vi "Python@SetVariable(Worker)__Parameter.vi"(1 "ParamterIn":string) -> (0 "ParamterOut":string)   [LabVIEW 2020]
panel:
  in  "Session":string(combo)
  in  "PythonName":string(combo) caption="PythonName="
  in  "Section":string(combo)
  in  "ParameterName":string(combo)
  in  "Confirm":bool
  # "Python@SetVariable(Worker) $Worker$Variable(,$section,PythonName=)"
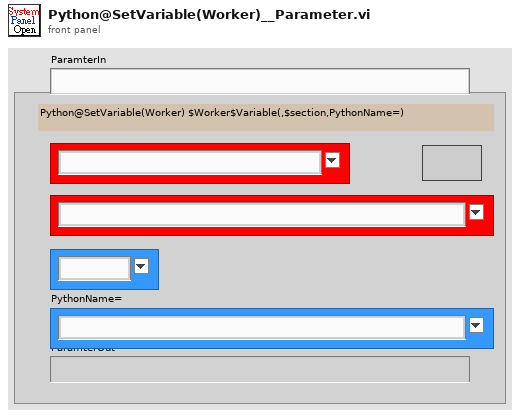
[diagram p1: front panel]
types:
  T1 = enum16{"Get", "Init", "Set", "Delete", "GetElement", "Inc", "Dec", "ReName"}
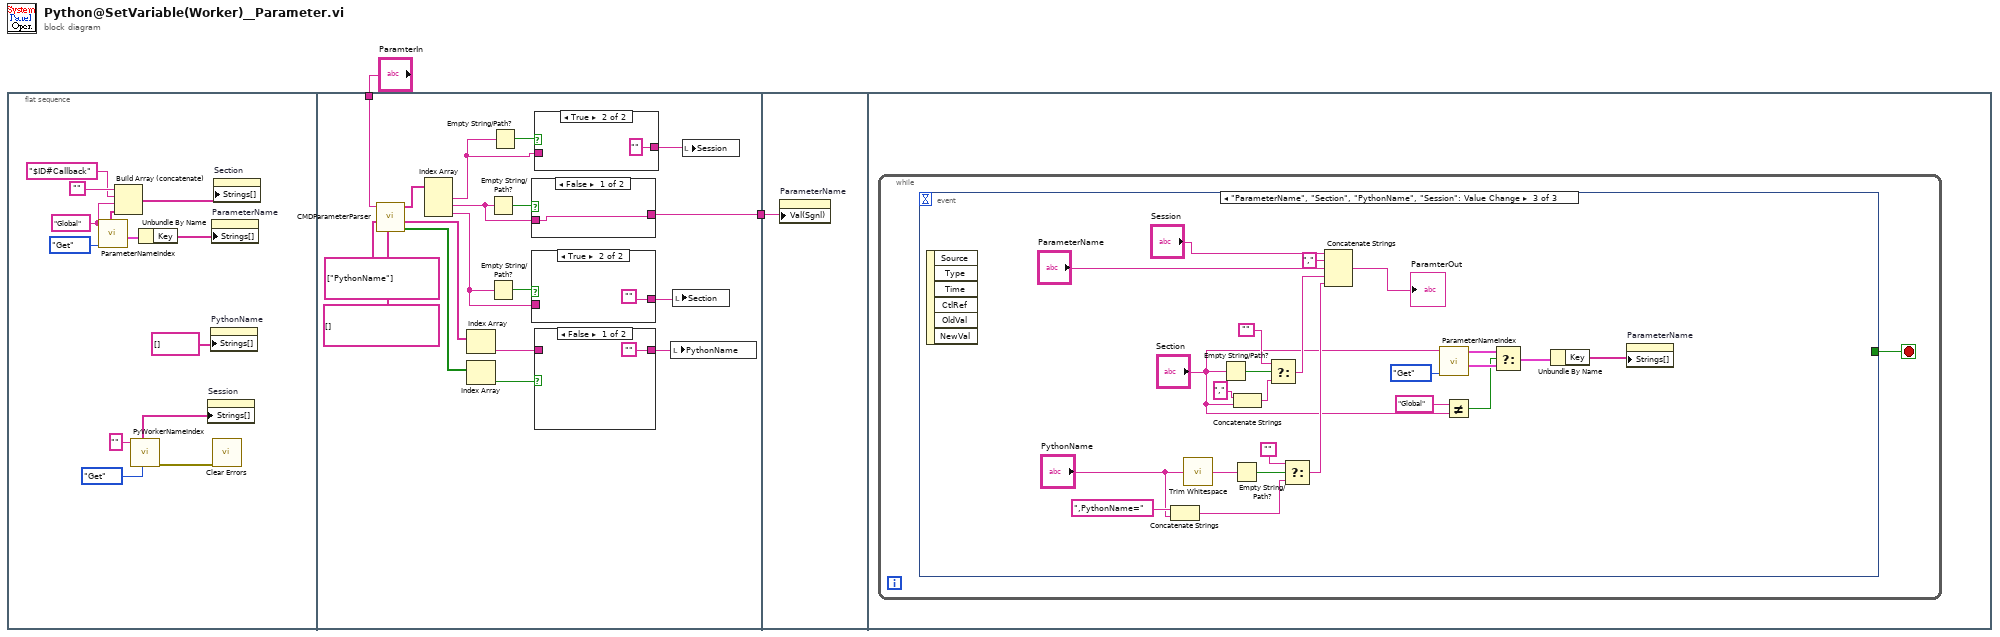
[diagram p0: block diagram]
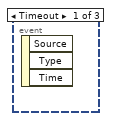
[diagram p6: hidden frame]
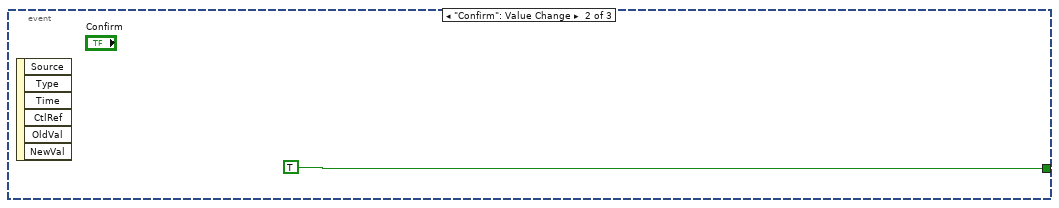
[diagram p7: hidden frame]
diagram:
  n1 = flat-sequence {
    tunnel: "ParamterIn" -> [w26]
    tunnel: [w32] -> w1
    tunnel: w1 -> [w42]
    frame #0 {
      w10 = "Global" ("VariableSection")
      n2 = call "ParameterNameIndex.vi"("OP"=T1."Get", "VariableSection"=w10) -> ("GlobalKeyValue"=w15:cluster{"Key":string[], "Value":string[]}, "SectionList"=w11:string[])  [unwired: 3 in, 5 out]
      n3 = Build Array (concatenate)("", "$ID#Callback" ("VariableSection"), w10, w11) -> (w9:string[])
      n4 = call "PyWorkerNameIndex.vi"("OP"=enum16{"Init", "Get", "Set"}."Get", "WrokerName"="" ("SessionIn")) -> ("error out"=w3:errorcluster, "PythonWorkerNameS"=w4:string[])  [unwired: 6 in, 2 out]
      n5 = Unbundle By Name(w15) -> ("Key"=w14:string[])
      n6 = property on="Session" class="CmbBox"("Strings[]"=w4) -> ()  [unwired: 2 in, 2 out]
      n7 = property on="PythonName" class="CmbBox"("Strings[]"=string[] [] ("Strings []")) -> ()  [unwired: 2 in, 2 out]
      n8 = property on="ParameterName" class="CmbBox"("Strings[]"=w14) -> ()  [unwired: 2 in, 2 out]
      n9 = call <vilib>:"Clear Errors.vi"("error in (no error)"=w3) -> ()  [unwired: 5 in, 2 out]
      n10 = property on="Section" class="CmbBox"("Strings[]"=w9) -> ()  [unwired: 2 in, 2 out]
    }
    frame #1 {
      n11 = call "CMDParameterParser.vi"("DeafultValues"=string[] [], "RequiredKeys"=string[] ["PythonName"], "CMDParameter"=w26) -> ("KeyFind?"=w22:bool[], "KeyValues"=w23:string[], "Input"=w27:string[])  [unwired: 6 in]
      n12 = Index Array(array=w27) -> (element #1=w18:string, element #2=w31:string, element #3=w28:string)  [unwired: 3 in]
      n13 = Index Array(array=w23) -> (element=w20:string)  [unwired: 1 in]
      n14 = Index Array(array=w22) -> (element=w21:bool)  [unwired: 1 in]
      n15 = Empty String/Path?(string/path=w31) -> (empty?=w33:bool)
      n16 = Empty String/Path?(string/path=w28) -> (empty?=w30:bool)
      n17 = Empty String/Path?(string/path=w18) -> (empty?=w17:bool)
      n18 = case shown="False" w33 {
        tunnel: w31 -> [w40 w41]
        tunnel: [w40 w41] -> w32
        frame False {
        }
        frame True {
        }
      }
      n19 = case shown="True" w30 {
        tunnel: w28 -> [w38 _]
        tunnel: [w38 ""] -> w29
        frame False {
        }
        frame True {
        }
      }
      n20 = case shown="True" w17 {
        tunnel: w18 -> [w34 _]
        tunnel: [w34 ""] -> w16
        frame False {
        }
        frame True {
        }
      }
      n21 = case shown="False" w21 {
        tunnel: w20 -> [_ w37]
        tunnel: ["" w37] -> w19
        frame False {
        }
        frame True {
        }
      }
      n22 = local write "PythonName"(w19) -> ()
      n23 = local write "Section"(w29) -> ()
      n24 = local write "Session"(w16) -> ()
    }
    frame #2 {
      n25 = property on="ParameterName" class="CmbBox"("Val(Sgnl)"=w42) -> ()  [unwired: 2 in, 2 out]
    }
    frame #3 {
      n26 = while {
        stop <- w43 stop-if-true
        n27 = event shown="[2] \"ParameterName\", \"Section\", \"PythonName\", \"Session\": Value Change" {
          selector: _ -> [_ _ _]
          dyn-events: _ -> [_ _ _]
          timeout: _ -> [_ _ _]
          tunnel: [_ TRUE _] -> w43
          event Timeout {
            n28 = event-data() -> ()  [unwired: 1 in, 3 out]
          }
          event "Confirm": Value Change {
            n29 = event-data() -> ()  [unwired: 1 in, 6 out]
          }
          event "ParameterName", "Section", "PythonName", "Session": Value Change {
            n30 = event-data() -> ()  [unwired: 1 in, 6 out]
            n31 = Concatenate Strings(",PythonName=" ("string"), "PythonName") -> (w55:string)
            n32 = call <vilib>:"Trim Whitespace.vi"("string"="PythonName") -> ("trimmed string"=w58:string)  [unwired: 1 in]
            n33 = Empty String/Path?(string/path="Section") -> (empty?=w64:bool)
            n34 = Empty String/Path?(string/path=w58) -> (empty?=w57:bool)
            n35 = Concatenate Strings("," ("string"), "Section") -> (w65:string)
            n36 = Select(t="", s=w64, f=w65) -> (s? t:f=w61:string)
            n37 = Select(t="", s=w57, f=w55) -> (s? t:f=w53:string)
            n38 = Concatenate Strings("Session", "," ("string"), "ParameterName", w61, w53) -> (→"ParamterOut":string)
            n39 = call "ParameterNameIndex.vi"("OP"=T1."Get", "VariableSection"="Section") -> ("GlobalKeyValue"=w51:cluster{"Key":string[], "Value":string[]}, "SectionKeyValue"=w52:cluster{"Key":string[], "Value":string[]})  [unwired: 3 in, 5 out]
            n40 = Not Equal?(x="Global", y="Section") -> (x != y?=w48:bool)
            n41 = Select(t=w52, s=w48, f=w51) -> (s? t:f=w47:cluster{"Key":string[], "Value":string[]})
            n42 = Unbundle By Name(w47) -> ("Key"=w63:string[])
            n43 = property on="ParameterName" class="CmbBox"("Strings[]"=w63) -> ()  [unwired: 2 in, 2 out]
          }
        }
      }
    }
  }
